vi "F-MaskFilterProcess.vi"() -> ()   [LabVIEW 2014]
doc: "Use this template to build a VI to use as a subVI."
uses:
  <vilib>/vision/NI_Vision_Development_Module.lvlib
panel:
  in  "v0":i16=60
  in  "u0":i16=128
  in  "D1":u16=30
  in  "D0":u16=15
  in  "Filter":T1(ring)=enum."INRF"
  out "|F(u,v)H(u,v)|":T2(plugin-control)
  out "g(x,y)":T2(plugin-control)
  out "IF(u,v)I":T2(plugin-control)
  out "f(x,y)":T2(plugin-control)
  # "1) low/high pass filter controlled by D0;\n2) Band pass/reject controlled by D0(low cut) and D1(high cut);\n3) Notch Filter controlled by (+/-u0,+/-v0) and D0;"
  # ":: MVi Framework V1.0 ::\nAuthor:Gaoke Yang\nEmail: gaoke.yang@yahoo.com\nWeb: www.mvicontrol.com\nCopyright (C) 2015, MVi Technologies All Rights Reserved"
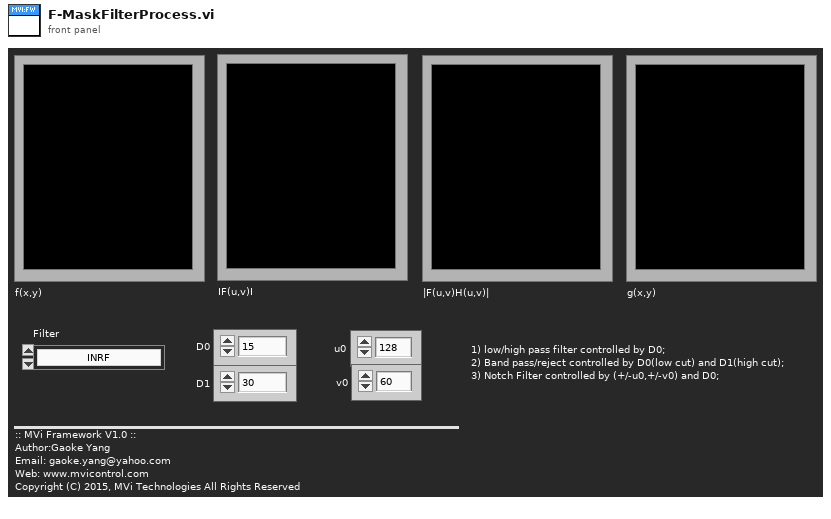
[diagram p1: front panel]
types:
  T1 = enum16{"ILPF", "IHPF", "IBPF", "IBRF", "INPF", "INRF"}
  T2 = typedef "IMAQ Image.ctl" = refnum<image>
  T3 = typedef "Image Type" = u32
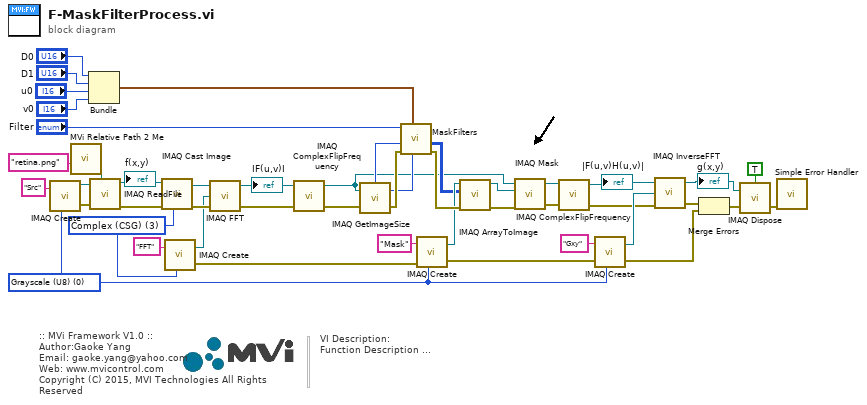
[diagram p0: block diagram]
diagram:
  w6 = T3 0 items=["Grayscale (U8)", "Grayscale (I16)", "Grayscale (SGL)", "Complex (CSG)", "RGB (U32)", "HSL (U32)", "RGB (U64)", "Grayscale (U16)"] ("Image Type")
  w16 = T3 3 items=["Grayscale (U8)", "Grayscale (I16)", "Grayscale (SGL)", "Complex (CSG)", "RGB (U32)", "HSL (U32)", "RGB (U64)", "Grayscale (U16)"] ("Image Type")
  # "VI Description:\nFunction Description ..."
  # ":: MVi Framework V1.0 ::\nAuthor:Gaoke Yang\nEmail: gaoke.yang@yahoo.com\nWeb: www.mvicontrol.com\nCopyright (C) 2015, MVI Technologies All Rights Reserved"
  n1 = call "IMAQ Create"("Image Name"="Src" ("name or relative path"), "Image Type"=w6) -> ("New Image"=w43:T2, "error out"=w42:errorcluster)  [unwired: 2 in, 1 out]
  n2 = call "MVi Relative Path 2 Me.vi"("Relative Path"="retina.png" ("name or relative path")) -> ("Appended Dir"=w39:path)  [unwired: 5 in, 1 out]
  n3 = Bundle("D0"="D0", "D1"="D1", "u0"="u0", "v0"="v0") -> (w1:cluster{"D0":u16, "D1":u16, "u0":i16, "v0":i16})  [unwired: 1 in]
  n4 = call "IMAQ ReadFile"("File Path"=w39, "error in (no error)"=w42, "Image"=w43) -> ("error out"=w36:errorcluster, "Image Out"=w35:T2)  [unwired: 4 in, 3 out]
  "f(x,y)" <- w35
  n5 = call "IMAQ Cast Image"("Image Type"=w16, "error in (no error)"=w36, "Image Src"=w35) -> ("error out"=w38:errorcluster, "Image Dst Out"=w34:T2)  [unwired: 7 in]
  n6 = call "IMAQ Create"("Image Name"="FFT" ("name or relative path"), "Image Type"=w16) -> ("New Image"=w33:T2, "error out"=w31:errorcluster)  [unwired: 2 in, 1 out]
  n7 = call "IMAQ FFT"("error in (no error)"=w38, "Image Dst"=w33, "Image Src"=w34) -> ("error out"=w28:errorcluster, "Image Dst Out"=w27:T2)  [unwired: 1 in]
  "IF(u,v)I" <- w27
  n8 = call "IMAQ ComplexFlipFrequency"("error in (no error)"=w28, "Image Src"=w27) -> ("error out"=w24:errorcluster, "Image Dst Out"=w11:T2)  [unwired: 2 in]
  n9 = call "IMAQ GetImageSize"("Image"=w11, "error in (no error)"=w24) -> ("Y Resolution"=w15:i32, "X Resolution"=w14:i32, "error out"=w23:errorcluster)  [unwired: 2 in]
  n10 = call "MaskFilters.vi"("ImgY"=w15, "FilterParam"=w1, "EorIn"=w23, "ImgX"=w14, "Filter"="Filter") -> ("ErrOut"=w22:errorcluster, "H(u,v)"=w12:u8[][])  [unwired: 5 in]
  n11 = call "IMAQ Create"("Image Name"="Mask" ("name or relative path"), "Image Type"=w6, "error in (no error)"=w31) -> ("New Image"=w17:T2, "error out"=w18:errorcluster)  [unwired: 1 in, 1 out]
  n12 = call "IMAQ ArrayToImage"("error in (no error)"=w22, "Image Pixels (U8)"=w12, "Image"=w17) -> ("error out"=w10:errorcluster, "Image Out"=w9:T2)  [unwired: 7 in]
  n13 = call "IMAQ Mask"("error in (no error)"=w10, "Image Mask"=w9, "Image Src"=w11) -> ("error out"=w8:errorcluster, "Image Dst Out"=w7:T2)  [unwired: 2 in]
  n14 = call "IMAQ ComplexFlipFrequency"("error in (no error)"=w8, "Image Src"=w7) -> ("error out"=w26:errorcluster, "Image Dst Out"=w25:T2)  [unwired: 2 in]
  "|F(u,v)H(u,v)|" <- w25
  n15 = call "IMAQ Create"("Image Name"="Gxy" ("name or relative path"), "Image Type"=w6, "error in (no error)"=w18) -> ("New Image"=w29:T2, "error out"=w19:errorcluster)  [unwired: 1 in, 1 out]
  n16 = call "IMAQ InverseFFT"("error in (no error)"=w26, "Image Dst"=w29, "Image Src"=w25) -> ("error out"=w21:errorcluster, "Image Dst Out"=w20:T2)  [unwired: 1 in]
  "g(x,y)" <- w20
  n17 = Merge Errors(w21, w19) -> (w37:errorcluster)
  n18 = call "IMAQ Dispose"("All Images? (No)"=TRUE, "Image"=w20, "error in (no error)"=w37) -> ("error out"=w44:errorcluster)  [unwired: 3 out]
  n19 = call <vilib>:"Simple Error Handler.vi"("error in (no error)"=w44) -> ()  [unwired: 1 in, 8 out]
